vi "test Anchor Object to Cluster Array.vi"(8 "error in (no error)":errorcluster, 11 "TestCase in":refnum<class "AnchorTests.lvclass">) -> (0 "error out":errorcluster, 3 "TestCase out":refnum<class "AnchorTests.lvclass">)   [LabVIEW 2014, in "AnchorTests.lvclass"]
uses:
  AnchorTests.lvclass
  <vilib>/addons/_JKI Toolkits/VI Tester/TestCase.llb/TestCase.lvclass
  SPLAT/Anchor/Anchor.lvclass
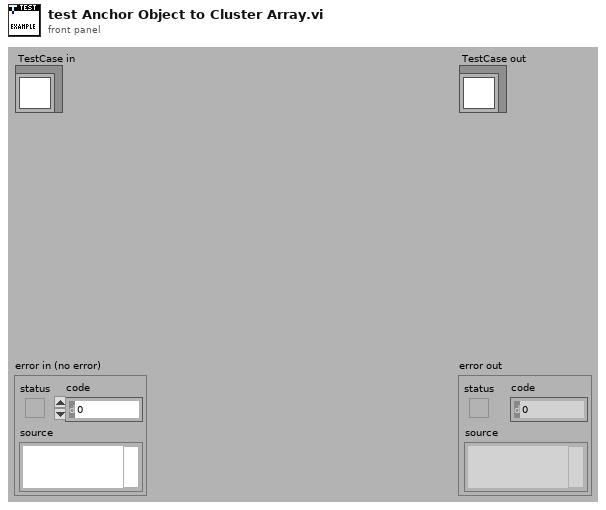
[diagram p1: front panel]
types:
  T1 = cluster{"AnchorID":dbl, "AnchorX":dbl, "AnchorY":dbl}[]
  T2 = cluster{"AnchorID":dbl, "AnchorX":dbl, "AnchorY":dbl}
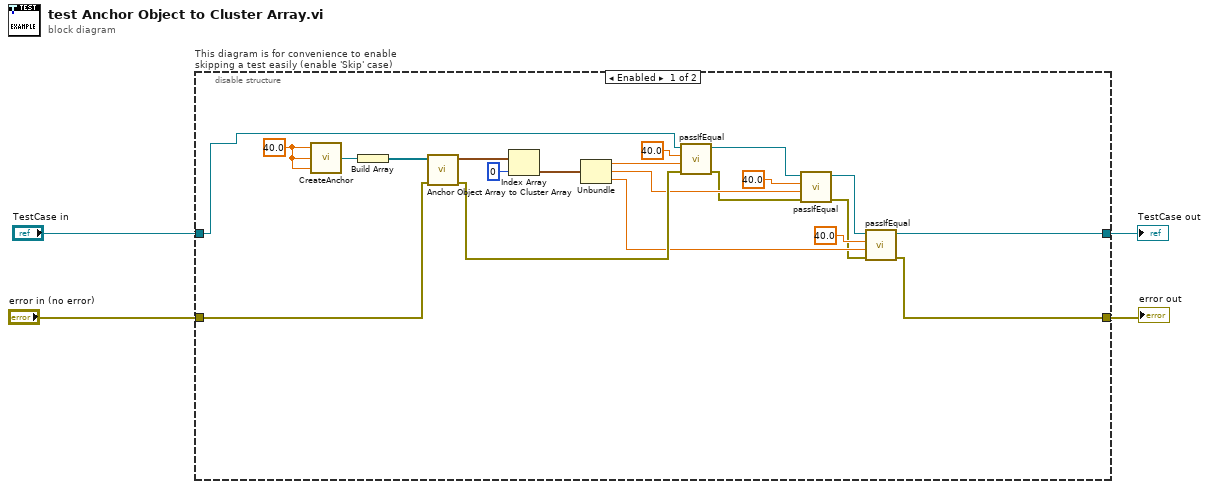
[diagram p0: block diagram]
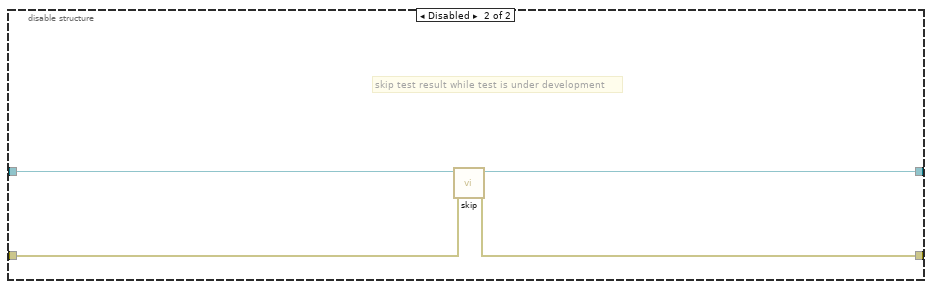
[diagram p2: hidden frame]
diagram:
  n1 = disable-structure "This diagram is for convenience to enable skipping a test easily (enable 'Skip' case)" shown="Enabled" {
    disable-tunnel: "TestCase in" -> [w15 w29]
    disable-tunnel: [w20 w27] -> w1
    disable-tunnel: [w21 w28] -> w3
    disable-tunnel: "error in (no error)" -> [w22 w26]
    frame Enabled {
      w25 = 40.0 ("Anchor ID")
      n2 = call "CreateAnchor.vi"("Anchor Y"=w25, "Anchor X"=w25, "Anchor ID"=w25) -> ("Anchor Out"=w24:refnum<class "Anchor.lvclass">)
      n3 = Build Array(w24) -> (w23:refnum<class "Anchor.lvclass">[])
      n4 = call "Anchor Object Array to Cluster Array.vi"("error in (no error)"=w22, "AnchorArray In"=w23) -> ("error out"=w13:errorcluster, "AnchorArray Out"=w19:T1)  [unwired: 8 in]
      n5 = Index Array(array=w19, index=0) -> (element=w17:T2)
      n6 = Unbundle(w17) -> ("AnchorID"=w16:dbl, "AnchorX"=w12:dbl, "AnchorY"=w11:dbl)
      n7 = call-dynamic "passIfEqual.vi"("error in (no error)"=w13, "y"=w16, "x"=40.0 ("Anchor ID"), "TestCase in"=w15) -> ("error out"=w6:errorcluster, "TestCase out"=w8:refnum<class "AnchorTests.lvclass">)  [unwired: 6 in]
      n8 = call-dynamic "passIfEqual.vi"("error in (no error)"=w6, "y"=w12, "x"=40.0 ("Anchor ID"), "TestCase in"=w8) -> ("error out"=w5:errorcluster, "TestCase out"=w7:refnum<class "AnchorTests.lvclass">)  [unwired: 6 in]
      n9 = call-dynamic "passIfEqual.vi"("error in (no error)"=w5, "y"=w11, "x"=40.0 ("Anchor ID"), "TestCase in"=w7) -> ("error out"=w21:errorcluster, "TestCase out"=w20:refnum<class "AnchorTests.lvclass">)  [unwired: 6 in]
    }
    frame Disabled {
      # "skip test result while test is under development"
      n10 = call <vilib>:"skip.vi"("error in (no error)"=w26, "TestCase in"=w29) -> ("error out"=w28:errorcluster, "TestCase out"=w27:refnum<class "AnchorTests.lvclass">)  [unwired: 8 in]
    }
  }
  "error out" <- w3
  "TestCase out" <- w1
